vi "macro_vecBuilder2x1FIll.vi"   [LabVIEW 2019, in "Trajectory_Library.lvlib"]
uses:
  Trajectory_Library.lvlib
  MatBuilder_Create.vi
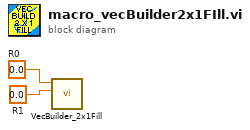
[diagram p0: block diagram]
diagram:
  w1 = 0.0  # R1
  w2 = 0.0  # R0
  n1 = call "VecBuilder_2x1Fill.vi"("R1"=w1, "R0"=w2) -> ()  [unwired: 9 in, 1 out]
